vi "MeasurePictureSize.vi"(8 "Split NxN":i32, 10 "image data":T1) -> (1 "N-width(Y)":i32, 2 "N-length(X)":i32)   [LabVIEW 2014]
uses:
  <vilib>/picture/picture.llb/imagedata.ctl
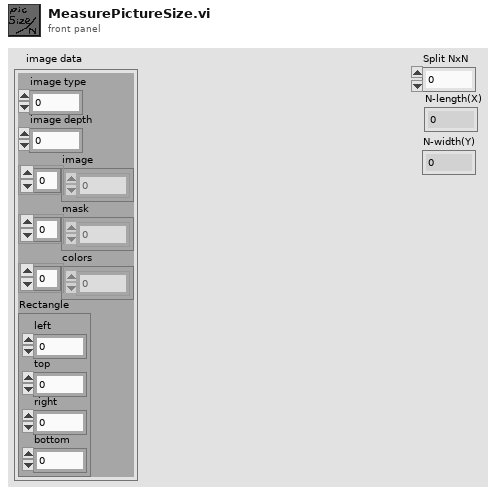
[diagram p1: front panel]
types:
  T1 = typedef "imagedata.ctl" = cluster{"image type":i32, "image depth":i32, "image":u8[], "mask":u8[], "colors":u32[], "Rectangle":cluster{"left":i16, "top":i16, "right":i16, "bottom":i16}}
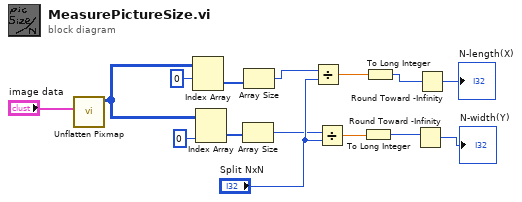
[diagram p0: block diagram]
diagram:
  n1 = call <vilib>:"Unflatten Pixmap.vi"("image data"="image data") -> ("24-bit pixmap"=w15:u32[][])  [unwired: 4 in, 6 out]
  n2 = Index Array(array=w15, index (row)=0) -> (element=w12:u32[])  [unwired: 1 in]
  n3 = Index Array(array=w15, index (col)=0 ("disabled index (col)")) -> (element=w11:u32[])  [unwired: 1 in]
  n4 = Array Size(array=w11) -> (size(s)=w8:i32)
  n5 = Array Size(array=w12) -> (size(s)=w10:i32)
  n6 = Divide(x=w10, y="Split NxN") -> (x/y=w6:dbl)
  n7 = Divide(x=w8, y="Split NxN") -> (x/y=w7:dbl)
  n8 = To Long Integer(number=w7) -> (32bit integer=w5:i32)
  n9 = To Long Integer(number=w6) -> (32bit integer=w4:i32)
  n10 = Round Toward -Infinity(1:w5) -> (0:→"N-width(Y)":i32)
  n11 = Round Toward -Infinity(1:w4) -> (0:→"N-length(X)":i32)
